vi "libdaq_adc_config_channel.vi"(0 "error in (no error)":errorcluster, 1 "device_name":string, 2 "module_name":string, 7 "channel":u8, 9 "range":T1(ring), 11 "couplemode":enum8{"DC", "AC"}(ring), 13 "refground":enum8{"RSE", "NRSE", "DIFF"}(ring)) -> (14 "error out":errorcluster, 15 "device_name":string, 16 "module_name":string)   [LabVIEW 2022 SP3, in "libdaqVI.lvlib"]
doc: "配置ADC模块的物理通道参数"
uses:
  libdaqVI.lvlib
  dll/daqlib.dll
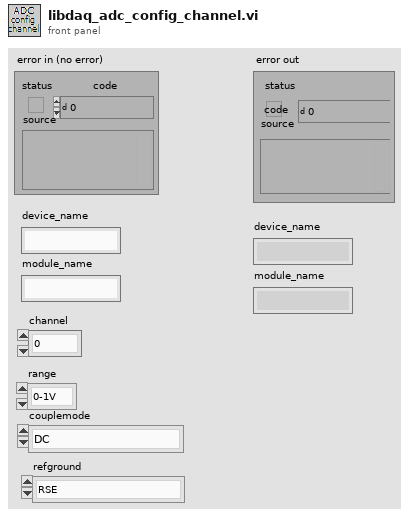
[diagram p1: front panel]
types:
  T1 = enum16{"0-1V", "0-2V", "0-2.5V", "0-5V", "0-10V", "±78.125mV", "±156.25mV", "±312.5mV", "±0.256V", "±0.512V", "±0.625V", "±1V", "±1.024V", "±1.25V", "±2V", "±2.048V", "±2.5V", "±4.096V", "±5.0V", "±10V", "0-20mA", "±20mA", "0-40mA", "±40mA"}
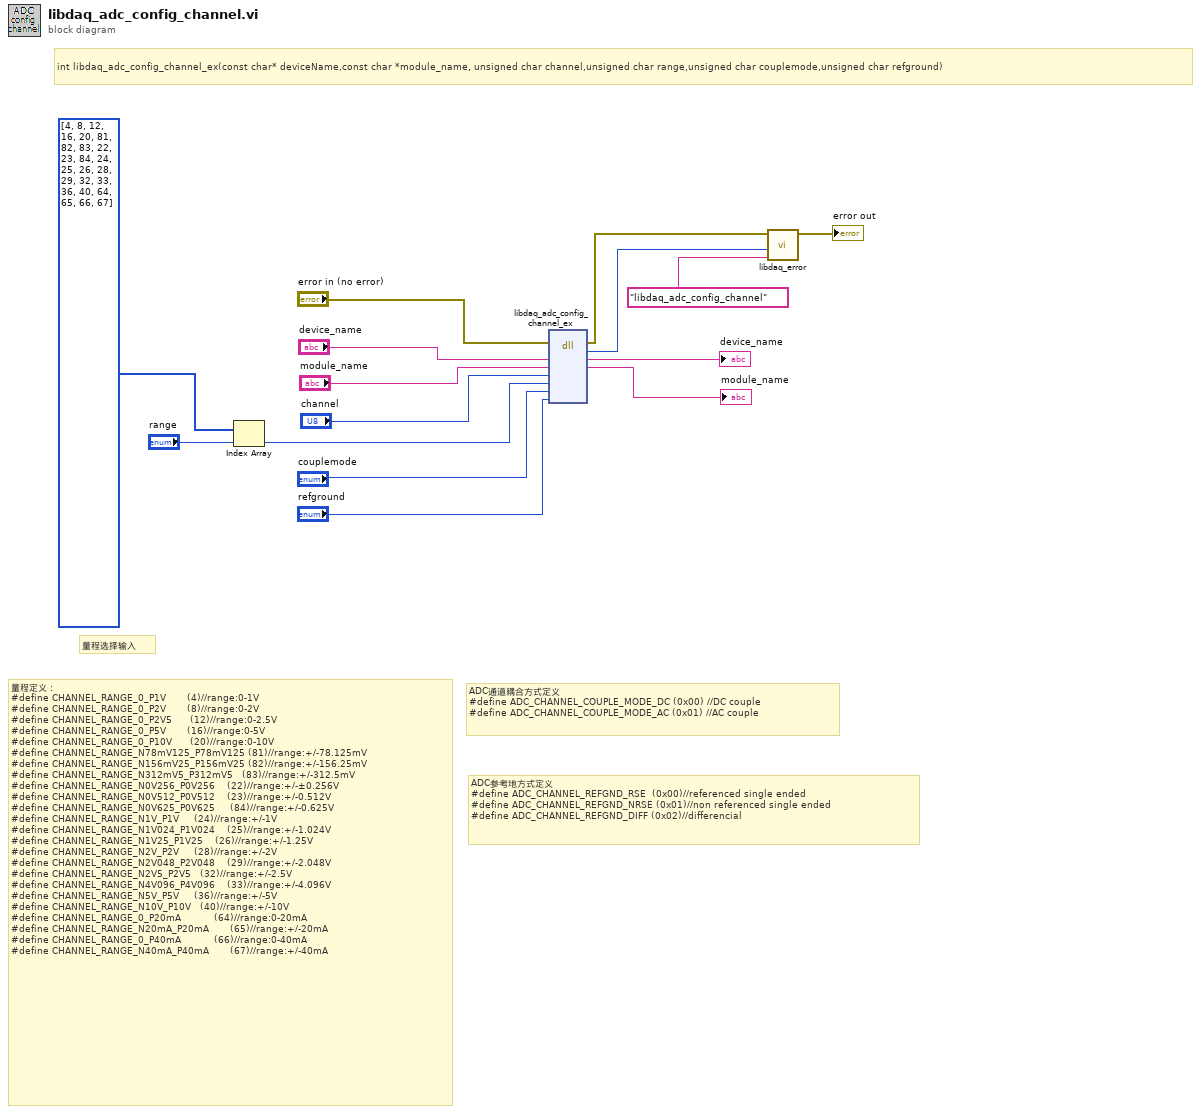
[diagram p0: block diagram]
diagram:
  # "ADC参考地方式定义\n#define ADC_CHANNEL_REFGND_RSE  (0x00)//referenced single ended\n#define ADC_CHANNEL_REFGND_NRSE (0x01)//non referenced single ended\n#define ADC_CHANNEL_REFGND_DIFF (0x02)//differencial"
  # "ADC通道耦合方式定义\n#define ADC_CHANNEL_COUPLE_MODE_DC (0x00) //DC couple\n#define ADC_CHANNEL_COUPLE_MODE_AC (0x01) //AC couple"
  # "量程定义：\n#define CHANNEL_RANGE_0_P1V     \t\t(4)//range:0-1V\n#define CHANNEL_RANGE_0_P2V     \t\t(8)//range:0-2V\n#define CHANNEL_RANGE_0_P2V5    \t\t(12)//range:0-2.5V\n#define CHANNEL_RANGE_0_P5V     \t\t(16)//range:0-5V\n#define CHANNEL_RANGE_0_P10V    \t\t(20)//range:0-10V\n#define CHANNEL_RANGE_N78mV125_P78mV125 (81)//range:+/-78.125mV\n#define CHANNEL_RANGE_N156mV25_P156mV25 (82)//range:+/-156.25mV\n#define CHANNEL_RANGE_N312mV5_P312mV5   (83)//range:+/-312.5mV\n#define CHANNEL_RANGE_N0V256_P0V256   \t(22)//range:+/-±0.256V\n#define CHANNEL_RANGE_N0V512_P0V512   \t(23)//range:+/-0.512V\n#define CHANNEL_RANGE_N0V625_P0V625     (84)//range:+/-0.625V\n#define CHANNEL_RANGE_N1V_P1V   \t\t(24)//range:+/-1V\n#define CHANNEL_RANGE_N1V024_P1V024   \t(25)//range:+/-1.024V\n#define CHANNEL_RANGE_N1V25_P1V25   \t(26)//range:+/-1.25V\n#define CHANNEL_RANGE_N2V_P2V   \t\t(28)//range:+/-2V\n#define CHANNEL_RANGE_N2V048_P2V048   \t(29)//range:+/-2.048V\n#define CHANNEL_RANGE_N2V5_P2V5 \t\t(32)//range:+/-2.5V\n#define CHANNEL_RANGE_N4V096_P4V096   \t(33)//range:+/-4.096V\n#define CHANNEL_RANGE_N5V_P5V   \t\t(36)//range:+/-5V\n#define CHANNEL_RANGE_N10V_P10V \t\t(40)//range:+/-10V\n#define CHANNEL_RANGE_0_P20mA           (64)//range:0-20mA\n#define CHANNEL_RANGE_N20mA_P20mA       (65)//range:+/-20mA\n#define CHANNEL_RANGE_0_P40mA           (66)//range:0-40mA\n#define CHANNEL_RANGE_N40mA_P40mA       (67)//range:+/-40mA"
  # "量程选择输入"
  # "int libdaq_adc_config_channel_ex(const char* deviceName,const char *module_name, unsigned char channel,unsigned char range,unsigned char couplemode,unsigned char refground)"
  n1 = Index Array(array=u8[] [4, 8, 12, 16, 20, 81, 82, 83, 22, 23, 84, 24, 25, 26, 28, 29, 32, 33, 36, 40, 64, 65, 66, 67], index="range") -> (element=w9:u8)
  n2 = dll-call lib="D:/Labview_projects/DAQ_USB3212/libdaqVI/dll/daqlib.dll" fn="libdaq_adc_config_channel_ex"(error in="error in (no error)", "device_name"="device_name", "module_name"="module_name", "channel"="channel", "range"=w9, "couplemode"="couplemode", "refground"="refground") -> (error out=w6:errorcluster, "return type"=w4:i32, "device_name"=→"device_name":string, "module_name"=→"module_name":string)  [unwired: 6 in, 1 out]
  n3 = call "libdaq_error.vi"("error source"="libdaq_adc_config_channel", "error code"=w4, "错误输入（无错误）"=w6) -> ("错误输出"=→"error out":errorcluster)  [unwired: 8 in]
